vi "Draw Marker Lines.vi"(6 "Type":T1, 8 "XY":cluster{"X":dbl, "Y":dbl}, 9 "Marker Options":T2={"Color"=16723218, "pen"={"Width"=2, "Style"=enum."Solid"}, "font"={"Font Name"="Arial", "Size"=16, "Strikeout?"=FALSE, "Italic?"=FALSE, "Underline?"=FALSE, "Outline?"=FALSE, "Shadow?"=FALSE, "Bold?"=FALSE, "FontColor"=0}, "caption"=""}, 10 "position":T3, 11 "picture":picture) -> (3 "new picture":picture)   [LabVIEW 2020, in "Graph Extensions.lvlib"]
doc: "Draw the appropriate line for markers, depending on the type"
uses:
  Graph Extensions.lvlib
  <vilib>/Utility/miscctls.llb/LVPoint32TypeDef.ctl
  controls/MarkerOptions.ctl
  controls/markerType.ctl
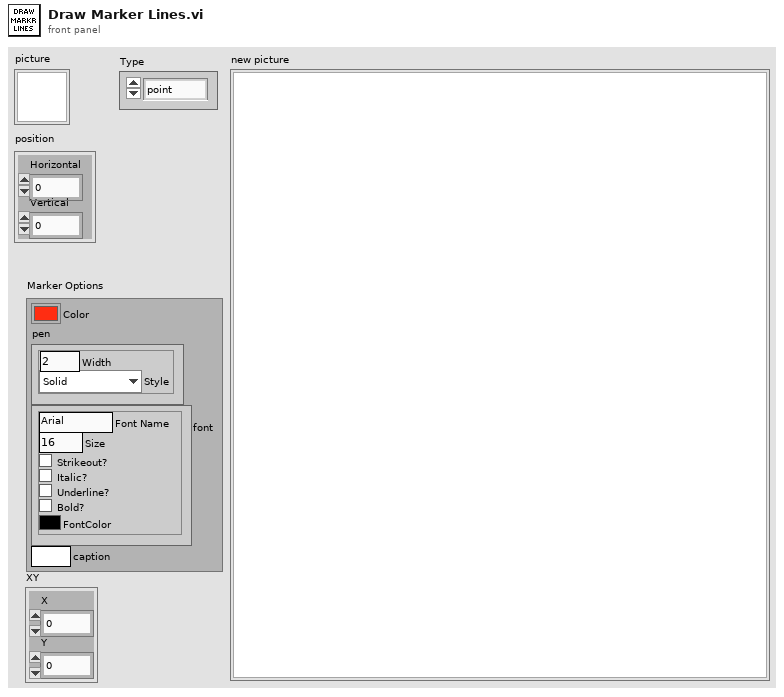
[diagram p1: front panel]
types:
  T1 = typedef "Graph Extensions.lvlib/markerType.ctl" = enum16{"point", "arrow", "horiz", "vert", "vert range", "horiz range", "box"}
  T2 = typedef "Graph Extensions.lvlib/MarkerOptions.ctl" = cluster{"Color":u32, "pen":cluster{"Width":u16, "Style":enum32{"Solid", "Dash", "Dot", "DashDot", "DashDotDot"}}, "font":cluster{"Font Name":string, "Size":i16, "Strikeout?":bool, "Italic?":bool, "Underline?":bool, "Outline?":bool, "Shadow?":bool, "Bold?":bool, "FontColor":u32}, "caption":string}
  T3 = typedef "LVPoint32TypeDef.ctl" = cluster{"Horizontal":i32, "Vertical":i32}
  T4 = enum32{"Solid", "Dash", "Dot", "DashDot", "DashDotDot"}
  T5 = cluster{"Font Name:":string, "Size":i16, "Strikeout?":bool, "Italic?":bool, "Underline?":bool, "Outline?":bool, "Shadow?":bool, "Bold?":bool}
  T6 = enum16{"User-specified Font", "Application Font", "System Font", "Dialog Font"}
  T7 = cluster{"Font Name":string, "Size":i16, "Strikeout?":bool, "Italic?":bool, "Underline?":bool, "Outline?":bool, "Shadow?":bool, "Bold?":bool, "FontColor":u32}
  T8 = cluster{"Width":u16, "Style":enum32{"Solid", "Dash", "Dot", "DashDot", "DashDotDot"}}
  T9 = cluster{"left":i16, "top":i16, "right":i16, "bottom":i16}
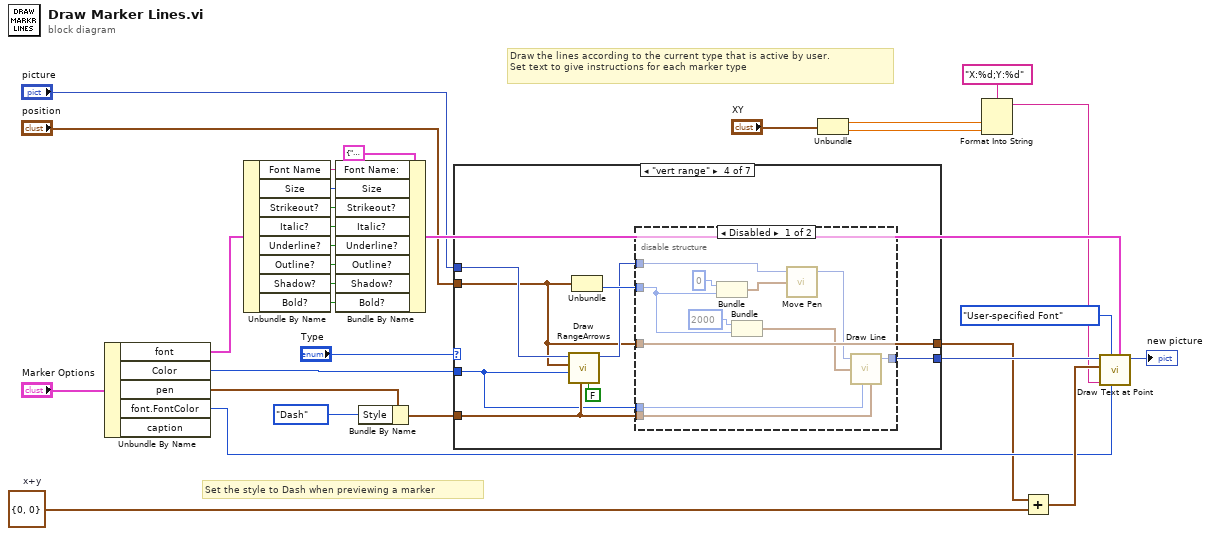
[diagram p0: block diagram]
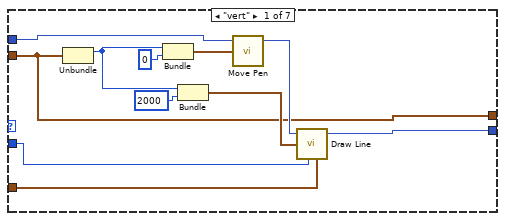
[diagram p2: hidden frame]
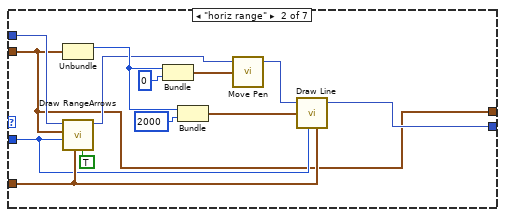
[diagram p3: hidden frame]
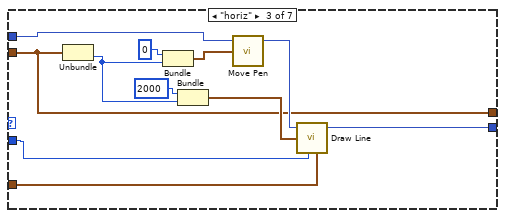
[diagram p4: hidden frame]
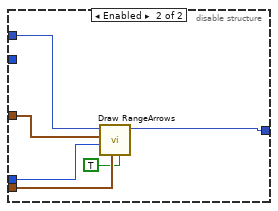
[diagram p5: hidden frame]
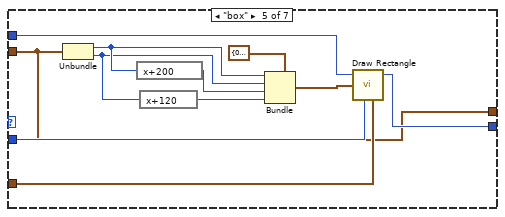
[diagram p6: hidden frame]
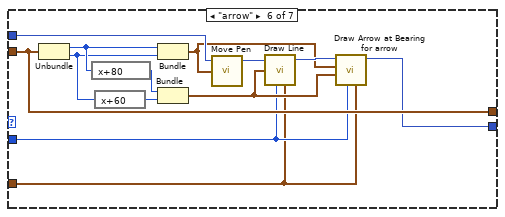
[diagram p7: hidden frame]
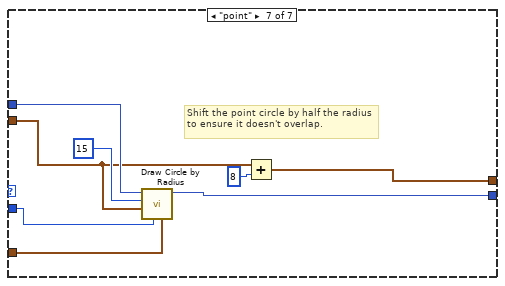
[diagram p8: hidden frame]
diagram:
  w7 = T3 {"Horizontal"=0, "Vertical"=0}  # x+y
  # "Set the style to Dash when previewing a marker"
  # "Draw the lines according to the current type that is active by user.\nSet text to give instructions for each marker type"
  n1 = Unbundle By Name("Marker Options") -> ("font"=w10:T7, "Color"=w15:u32, "pen"=w13:T8, "font.FontColor"=w26:u32)  [unwired: 1 out]
  n2 = Unbundle By Name(w10) -> ("Font Name"=w24:string, "Size"=w23:i16, "Strikeout?"=w22:bool, "Italic?"=w21:bool, "Underline?"=w20:bool, "Outline?"=w19:bool, "Shadow?"=w18:bool, "Bold?"=w17:bool)
  n3 = Bundle By Name(cluster=T5 {"Font Name:"="", "Size"=12, "Strikeout?"=FALSE, "Italic?"=FALSE, "Underline?"=FALSE, "Outline?"=FALSE, "Shadow?"=FALSE, "Bold?"=FALSE} ("[user-specified font]"), "Font Name:"=w24, "Size"=w23, "Strikeout?"=w22, "Italic?"=w21, "Underline?"=w20, "Outline?"=w19, "Shadow?"=w18, "Bold?"=w17) -> (w16:T5)
  n4 = Bundle By Name(cluster=w13, "Style"=T4."Dash") -> (w12:T8)
  n5 = case shown="\"vert range\"" "Type" {
    tunnel: "position" -> [w32 w44 w59 w67 w91 w114 w117]
    tunnel: [w40 w53 w65 w74 w99 w106 w122] -> w29
    tunnel: "picture" -> [w35 w48 w56 w69 w101 w113 w118]
    tunnel: w15 -> [w34 w45 w58 w70 w100 w104 w121]
    tunnel: w12 -> [w33 w46 w57 w71 w92 w102 w119]
    tunnel: [w32 w44 w59 w67 w91 w114 w115] -> w11
    frame "vert" {
      n6 = Unbundle(w32) -> ("Horizontal"=w42:i32)  [unwired: 1 out]
      n7 = Bundle("Horizontal"=w42, "top"=i16 0) -> (w36:cluster{"Horizontal":i32, "top":i16})  [unwired: 1 in]
      n8 = Bundle("Horizontal"=w42, "top"=i16 2000) -> (w41:cluster{"Horizontal":i32, "top":i16})  [unwired: 1 in]
      n9 = call <vilib>:"Move Pen.vi"("new position"=w36, "picture"=w35) -> ("new picture"=w39:picture)  [unwired: 3 in]
      n10 = call <vilib>:"Draw Line.vi"("picture"=w39, "end point"=w41, "color(black)"=w34, "pen"=w33) -> ("new picture"=w40:picture)  [unwired: 5 in]
    }
    frame "horiz range" {
      n11 = Unbundle(w44) -> ("Horizontal"=w55:i32)  [unwired: 1 out]
      n12 = call "Draw RangeArrows.vi"("Vertical"=TRUE, "pen"=w46, "Color"=w45, "position"=w44, "picture"=w48) -> ("new picture"=w47:picture)  [unwired: 6 in]
      n13 = Bundle("Horizontal"=w55, "top"=i16 0) -> (w49:cluster{"Horizontal":i32, "top":i16})  [unwired: 1 in]
      n14 = Bundle("Horizontal"=w55, "top"=i16 2000) -> (w54:cluster{"Horizontal":i32, "top":i16})  [unwired: 1 in]
      n15 = call <vilib>:"Move Pen.vi"("new position"=w49, "picture"=w47) -> ("new picture"=w52:picture)  [unwired: 3 in]
      n16 = call <vilib>:"Draw Line.vi"("picture"=w52, "end point"=w54, "color(black)"=w45, "pen"=w46) -> ("new picture"=w53:picture)  [unwired: 5 in]
    }
    frame "horiz" {
      n17 = Unbundle(w59) -> ("Vertical"=w61:i32)  [unwired: 1 out]
      n18 = Bundle("top"=i16 0, "Vertical"=w61) -> (w63:cluster{"top":i16, "Vertical":i32})  [unwired: 1 in]
      n19 = Bundle("top"=i16 2000, "Vertical"=w61) -> (w66:cluster{"top":i16, "Vertical":i32})  [unwired: 1 in]
      n20 = call <vilib>:"Move Pen.vi"("new position"=w63, "picture"=w56) -> ("new picture"=w64:picture)  [unwired: 3 in]
      n21 = call <vilib>:"Draw Line.vi"("picture"=w64, "end point"=w66, "color(black)"=w58, "pen"=w57) -> ("new picture"=w65:picture)  [unwired: 5 in]
    }
    frame "vert range" {
      n22 = call "Draw RangeArrows.vi"("Vertical"=FALSE, "pen"=w71, "Color"=w70, "position"=w67, "picture"=w69) -> ("new picture"=w68:picture)  [unwired: 6 in]
      n23 = Unbundle(w67) -> ("Vertical"=w73:i32)  [unwired: 1 out]
      n24 = disable-structure shown="Disabled" {
        disable-tunnel: [w83 w86] -> w74
        disable-tunnel: w73 -> [w79 _]
        disable-tunnel: w71 -> [w77 w88]
        disable-tunnel: w70 -> [w76 w87]
        disable-tunnel: w68 -> [w75 w90]
        disable-tunnel: w67 -> [_ w89]
        frame Disabled {
          n25 = Bundle("top"=i16 0, "Vertical"=w79) -> (w81:cluster{"top":i16, "Vertical":i32})  [unwired: 1 in]
          n26 = Bundle("top"=i16 2000, "Vertical"=w79) -> (w84:cluster{"top":i16, "Vertical":i32})  [unwired: 1 in]
          n27 = call <vilib>:"Move Pen.vi"("new position"=w81, "picture"=w75) -> ("new picture"=w82:picture)  [unwired: 3 in]
          n28 = call <vilib>:"Draw Line.vi"("picture"=w82, "end point"=w84, "color(black)"=w76, "pen"=w77) -> ("new picture"=w83:picture)  [unwired: 5 in]
        }
        frame Enabled {
          n29 = call "Draw RangeArrows.vi"("Vertical"=TRUE, "pen"=w88, "Color"=w87, "position"=w89, "picture"=w90) -> ("new picture"=w86:picture)  [unwired: 6 in]
        }
      }
    }
    frame "box" {
      n30 = Unbundle(w91) -> ("Horizontal"=w97:i32, "Vertical"=w94:i32)
      n31 = expression code="x+200"(w97) -> (w96:i32)
      n32 = expression code="x+120"(w94) -> (w93:i32)
      n33 = Bundle(cluster=T9 {"left"=0, "top"=0, "right"=0, "bottom"=0} ("rect"), "left"=w97, "top"=w94, "right"=w96, "bottom"=w93) -> (w98:T9)
      n34 = call <vilib>:"Draw Rectangle.vi"("picture"=w101, "rect"=w98, "color(black)"=w100, "pen"=w92) -> ("new picture"=w99:picture)  [unwired: 5 in]
    }
    frame "arrow" {
      n35 = Unbundle(w114) -> ("Horizontal"=w108:i32, "Vertical"=w107:i32)
      n36 = expression code="x+80"(w108) -> (w110:i32)
      n37 = expression code="x+60"(w107) -> (w109:i32)
      n38 = Bundle("Horizontal"=w108, "Vertical"=w107) -> (w103:cluster{"Horizontal":i32, "Vertical":i32})  [unwired: 1 in]
      n39 = Bundle("Horizontal"=w110, "Vertical"=w109) -> (w105:cluster{"Horizontal":i32, "Vertical":i32})  [unwired: 1 in]
      n40 = call <vilib>:"Move Pen.vi"("new position"=w103, "picture"=w113) -> ("new picture"=w112:picture)  [unwired: 3 in]
      n41 = call <vilib>:"Draw Line.vi"("picture"=w112, "end point"=w105, "color(black)"=w104, "pen"=w102) -> ("new picture"=w111:picture)  [unwired: 5 in]
      n42 = call "Draw Arrow at Bearing for arrow.vi"("pen"=w102, "color(black)"=w104, "P2"=w105, "P1"=w103, "new picture in"=w111) -> ("new picture out"=w106:picture)  [unwired: 6 in]
    }
    frame "point" {
      # "Shift the point circle by half the radius to ensure it doesn't overlap."
      n43 = call <vilib>:"Draw Circle by Radius.vi"("pen"=w119, "color(black)"=w121, "pixel center"=w117, "radius"=i16 15, "picture"=w118) -> ("new picture"=w122:picture)  [unwired: 6 in]
      n44 = Add(x=w117, y=8 ("Horizontal")) -> (x+y=w115:T3)
    }
  }
  n45 = Unbundle("XY") -> ("X"=w5:dbl, "Y"=w4:dbl)
  n46 = Format Into String(format string="X:%d;Y:%d", w5, w4) -> (resulting string=w2:string)  [unwired: 2 in, 1 out]
  n47 = Add(x=w11, y=w7) -> (x+y=w31:T3)
  n48 = call <vilib>:"Draw Text at Point.vi"("[user-specified font]"=w16, "text color(black)"=w26, "desired font(Application)"=T6."User-specified Font", "text"=w2, "origin"=w31, "picture"=w29) -> ("new picture"=→"new picture":picture)  [unwired: 4 in, 1 out]
